vi "Get Connections Impl.vi"(4 "pin type":T1, 6 "site":i32, 8 "error in":errorcluster, 9 "instrument":refnum<class "IInstrument.lvclass">, 10 "pin or relay names":string[](array[string]), 11 "session reservation in":refnum<class "Session Reservation.lvclass">) -> (0 "error out":errorcluster, 2 "connections":T2[](array[typedef]), 3 "session reservation out":refnum<class "Session Reservation.lvclass">)   [LabVIEW 2020, in "MeasurementLink Session Management.lvlib" / "Session Reservation.lvclass"]
uses:
  Session Reservation.lvclass
  Session Reservation.lvclass/Session Reservation.ctl
  Connection Map/Connection Map.lvclass
  MeasurementLink Measurement Server/Helpers/Error Strings Global Internal.vi
  MeasurementLink Instrument/IInstrument/IInstrument.lvclass
  Connection.ctl
  Connection with Session.ctl
  Pin Type.ctl
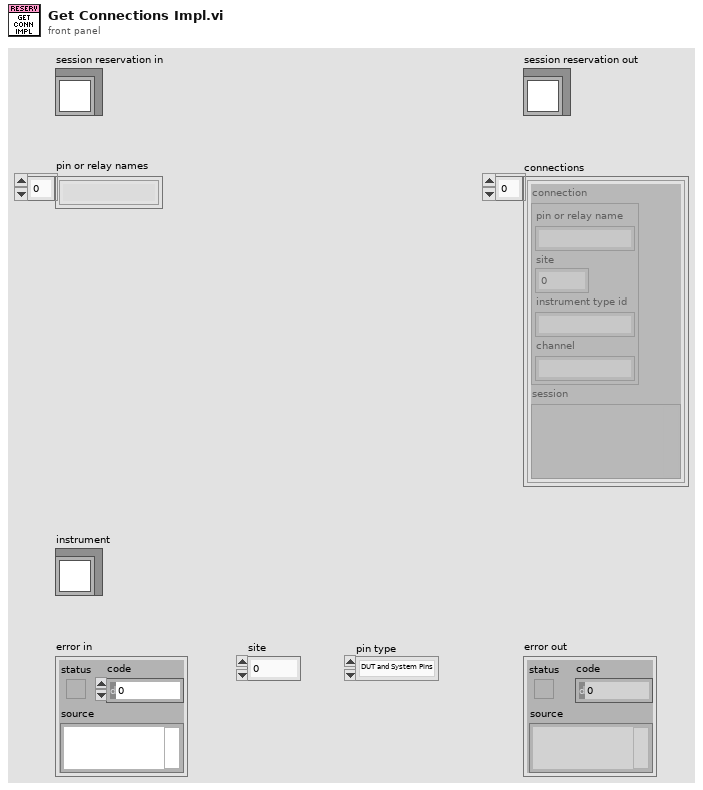
[diagram p1: front panel]
types:
  T1 = typedef "MeasurementLink Session Management.lvlib/Session Reservation.lvclass/Pin Type.ctl" = enum16{"DUT and System Pins", "System Pins"}
  T2 = typedef "MeasurementLink Session Management.lvlib/Session Reservation.lvclass/Connection with Session.ctl" = cluster{"connection":T3, "session":variant}
  T3 = typedef "MeasurementLink Session Management.lvlib/Session Reservation.lvclass/Connection.ctl" = cluster{"pin or relay name":string, "site":i32, "instrument type id":string, "channel":string}
  T4 = typedef "MeasurementLink Session Management.lvlib/Session Reservation.lvclass/Data.ctl" = cluster{"session and driver infos":T5[], "pin or relay names":string[], "connection map":refnum<class "Connection Map.lvclass">, "pin map context":T9, "reservation observer":refnum<class "IReservationObserver.lvclass">, "dvr valid":bool}
  T5 = typedef "MeasurementLink Session Management.lvlib/Session Reservation.lvclass/Session and Driver Info.ctl" = cluster{"session info":T6, "session":variant, "instrument":refnum<class "IInstrument.lvclass">}
  T6 = typedef "MeasurementLink Session Management Client.lvlib/ni_measurementlink_sessionmanagement_v1_SessionInformation.ctl" = cluster{"session":T7, "resource_name":string, "channel_list":string, "instrument_type_id":string, "session_exists":bool, "channel_mappings":T8[]}
  T7 = typedef "MeasurementLink Session Management Client.lvlib/nidevice_grpc_Session.ctl" = cluster{"name":string}
  T8 = typedef "MeasurementLink Session Management Client.lvlib/ni_measurementlink_sessionmanagement_v1_ChannelMapping.ctl" = cluster{"pin_or_relay_name":string, "site":i32, "channel":string}
  T9 = typedef "MeasurementLink Session Management Client.lvlib/ni_measurementlink_PinMapContext.ctl" = cluster{"pin_map_id":string, "sites":i32[]}
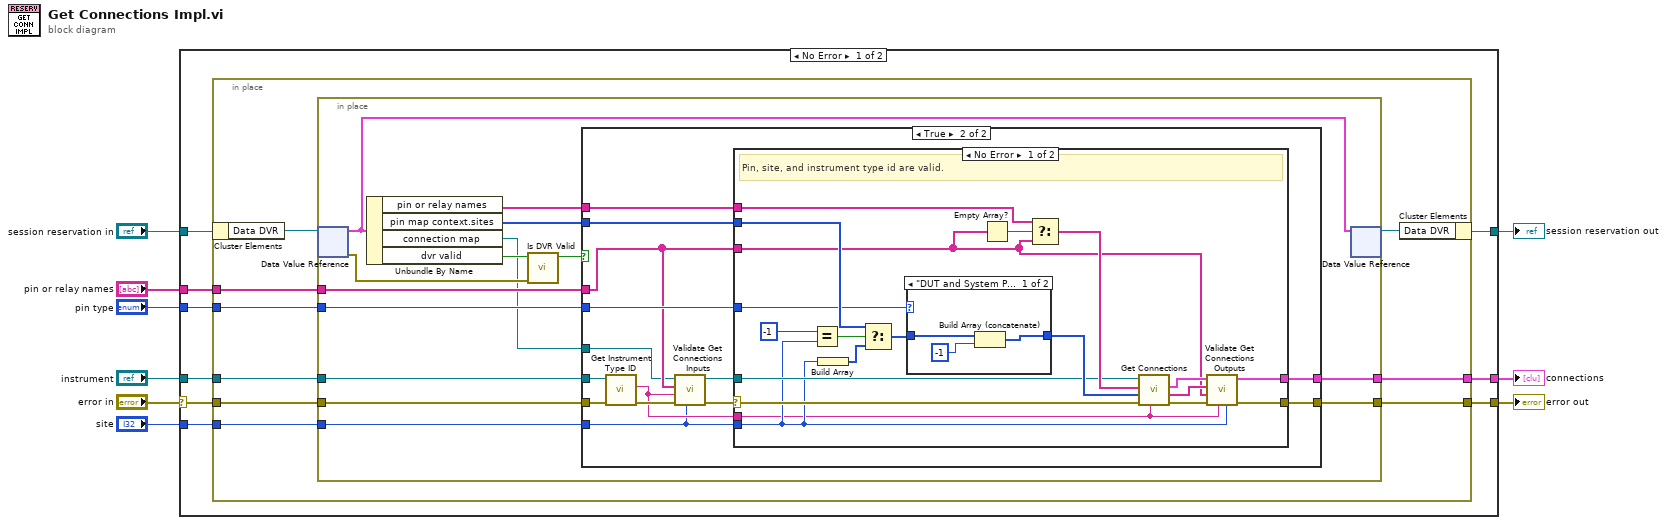
[diagram p0: block diagram]
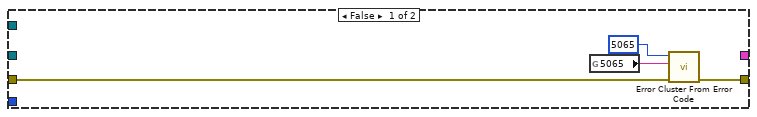
[diagram p2: hidden frame]
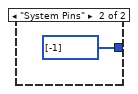
[diagram p3: hidden frame]
diagram:
  n1 = case shown="No Error" "error in" {
    selector: "error in" -> [w15 w86]
    tunnel: [w14 w86] -> w6
    tunnel: "session reservation in" -> [w12 w85]
    tunnel: "pin or relay names" -> [w18 _]
    tunnel: "site" -> [w17 _]
    tunnel: "instrument" -> [w16 _]
    tunnel: [w13 _] -> w4
    tunnel: [w11 w85] -> w2
    tunnel: "pin type" -> [w10 _]
    frame No Error {
      n2 = in-place {
        in-place-border: w18 -> [w27]
        in-place-border: w17 -> [w26]
        in-place-border: w16 -> [w25]
        in-place-border: w15 -> [w24]
        in-place-border: [w23] -> w14
        in-place-border: [w22] -> w13
        in-place-border: w10 -> [w19]
        n3 = in-place-cluster #1(w12) -> ("Data DVR"=w21:refnum<data-value>)
        n4 = in-place {
          in-place-border: w27 -> [w41]
          in-place-border: w26 -> [w40]
          in-place-border: w25 -> [w39]
          in-place-border: w24 -> [w38]
          in-place-border: [w37] -> w23
          in-place-border: [w36] -> w22
          in-place-border: w19 -> [w30]
          n5 = in-place-dvr #2(w21) -> (w31:T4, w33:errorcluster)
          n6 = Unbundle By Name(w31) -> ("pin or relay names"=w35:string[], "pin map context.sites"=w34:i32[], "connection map"=w28:refnum<class "Connection Map.lvclass">, "dvr valid"=w29:bool)
          n7 = call "Is DVR Valid.vi"("dvr error in"=w33, "dvr valid"=w29) -> ("dvr valid"=w32:bool)  [unwired: 9 in]
          n8 = case shown="True" w32 {
            tunnel: w41 -> [_ w48]
            tunnel: w40 -> [_ w47]
            tunnel: w39 -> [_ w59]
            tunnel: w38 -> [w43 w58]
            tunnel: [w42 w57] -> w37
            tunnel: [_ w56] -> w36
            tunnel: w35 -> [_ w55]
            tunnel: w34 -> [_ w54]
            tunnel: w30 -> [_ w53]
            tunnel: w28 -> [_ w46]
            frame False {
              n9 = global read "Error Strings Global Internal.vi" "5065"() -> (w45:string)
              n10 = call <vilib>:"Error Cluster From Error Code.vi"("error in (no error)"=w43, "error message (\"\")"=w45, "error code (0)"=5065) -> ("error out"=w42:errorcluster)  [unwired: 6 in]
            }
            frame True {
              n11 = call-dynamic "Get Instrument Type ID.vi"("error in (no error)"=w58, "instrument in"=w59) -> ("error out"=w52:errorcluster, "instrument type id"=w51:string)  [unwired: 7 in, 1 out]
              n12 = call "Validate Get Connections Inputs.vi"("site"=w47, "error in"=w52, "instrument type id"=w51, "pin or relay names"=w48, "connection map"=w46) -> ("error out"=w50:errorcluster, "connection map out"=w49:refnum<class "Connection Map.lvclass">)  [unwired: 5 in]
              n13 = case shown="No Error" w50 {
                selector: w50 -> [w69 w84]
                tunnel: [w66 w84] -> w57
                tunnel: [w62 _] -> w56
                tunnel: w55 -> [w75 _]
                tunnel: w54 -> [w73 _]
                tunnel: w53 -> [w70 _]
                tunnel: w51 -> [w64 _]
                tunnel: w49 -> [w68 _]
                tunnel: w48 -> [w60 _]
                tunnel: w47 -> [w65 _]
                frame No Error {
                  # "Pin, site, and instrument type id are valid."
                  n14 = Equal?(x=-1, y=w65) -> (x = y?=w78:bool)
                  n15 = Build Array(w65) -> (w79:i32[])
                  n16 = Select(t=w73, s=w78, f=w79) -> (s? t:f=w72:i32[])
                  n17 = case shown="\"DUT and System Pins\"" w70 {
                    tunnel: w72 -> [w81 _]
                    tunnel: [w80 i32[] [-1] ("sites")] -> w71
                    frame "DUT and System Pins" {
                      n18 = Build Array (concatenate)(w81, -1 ("x")) -> (w80:i32[])
                    }
                    frame "System Pins" {
                    }
                  }
                  n19 = Empty Array?(array=w60) -> (empty?=w74:bool)
                  n20 = Select(t=w75, s=w74, f=w60) -> (s? t:f=w76:string[])
                  n21 = call "Get Connections.vi"("instrument type id"=w64, "error in"=w69, "sites"=w71, "pin or relay names"=w76, "connection map in"=w68) -> ("error out"=w67:errorcluster, "pin or relay names found"=w61:string[], "connections"=w63:T2[])  [unwired: 3 in, 1 out]
                  n22 = call "Validate Get Connections Outputs.vi"("site"=w65, "instrument type id"=w64, "error in"=w67, "pin or relay names"=w60, "pin or relay names found"=w61, "connections in"=w63) -> ("error out"=w66:errorcluster, "connections out"=w62:T2[])  [unwired: 4 in]
                }
                frame Error {
                  # "Pin, site, or instrument type not in connections map."
                }
              }
            }
          }
          n23 = in-place-dvr #2(w31) -> (w20:refnum<data-value>)  [unwired: 1 out]
        }
        n24 = in-place-cluster #1("Data DVR"=w20) -> (w11:refnum<class "Session Reservation.lvclass">)
      }
    }
    frame Error {
    }
  }
  "error out" <- w6
  "connections" <- w4
  "session reservation out" <- w2
